vi "Do.vi"(8 "error in (no error)":errorcluster, 10 "Actor in":refnum<class "Actor.lvclass">, 11 "Send Packets Msg in":refnum<class "Send Packets Msg.lvclass">) -> (0 "error out":errorcluster, 2 "Actor out":refnum<class "Actor.lvclass">)   [LabVIEW 2021, in "Echo Broadcast Test With Server Manager.lvlib" / "Send Packets Msg.lvclass"]
doc: "(<B>Filename</B>: Actor Framework.lvlib:Message.lvclass:Do.vi)\n\nDefines what a message does when it is received by an actor. Generally, a message instructs an actor to invoke one of its methods. By default, this method does nothing. A child class must override it to define behavior. Create a child class by using the Actor Framework Message Maker dialog box."
uses:
  Send Packets Msg.lvclass
  <vilib>/ActorFramework/Actor/Actor.lvclass
  WS Test Server Subscriber/WS Test Server Subscriber.lvclass
  C:/Program Files/National Instruments/LabVIEW 2021/vi.lib/ActorFramework/Actor/Actor.lvclass
  Send Packets Msg.lvclass/Send Packets Msg.ctl
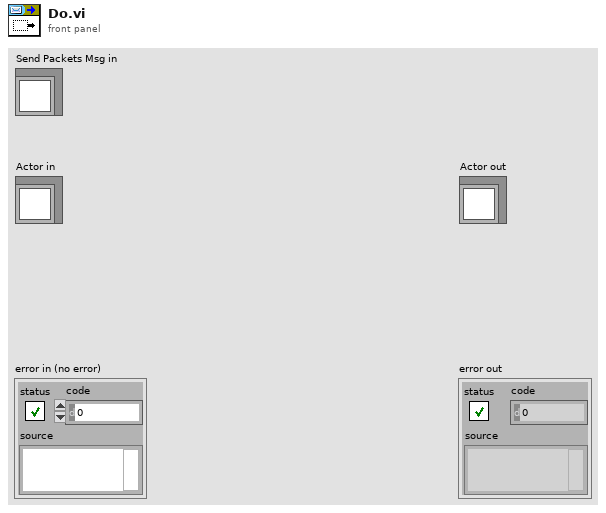
[diagram p1: front panel]
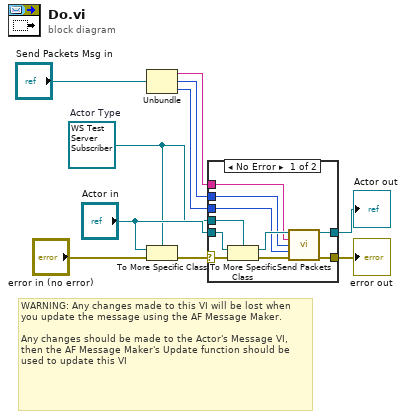
[diagram p0: block diagram]
diagram:
  w5 = refnum<class "WS Test Server Subscriber.lvclass"> refnum  # Actor Type
  # "WARNING: Any changes made to this VI will be lost when you update the message using the AF Message Maker.\n\nAny changes should be made to the Actor's Message VI, then the AF Message Maker's Update function should be used to update this VI"
  n1 = Unbundle("Send Packets Msg in") -> (w4:string, w3:i32, w2:i32)
  n2 = To More Specific Class(target class=w5, reference="Actor in", error in="error in (no error)") -> (error out=w9:errorcluster)  [unwired: 1 out]
  n3 = case shown="No Error" w9 {
    selector: w9 -> [w20 w22]
    tunnel: [w15 w22] -> w8
    tunnel: [w14 w21] -> w7
    tunnel: "Actor in" -> [w19 w21]
    tunnel: w5 -> [w18 _]
    tunnel: w4 -> [w13 _]
    tunnel: w3 -> [w12 _]
    tunnel: w2 -> [w11 _]
    frame No Error {
      n4 = To More Specific Class ("Actor Cast")(target class=w18, reference=w19, error in=w20) -> (specific class reference=w17:refnum<class "WS Test Server Subscriber.lvclass">, error out=w16:errorcluster)
      n5 = call "Send Packets.vi"("WS Test Server Subscriber in"=w17, "Data To Send"=w13, "Number of Packets"=w12, "Send Period (ms)"=w11, "error in (no error)"=w16) -> ("WS Test Server Subscriber out"=w14:refnum<class "WS Test Server Subscriber.lvclass">, "error out"=w15:errorcluster)  [unwired: 9 in]
    }
    frame Error {
    }
  }
  "error out" <- w8
  "Actor out" <- w7
